vi "format_console_string.vi"(8 "error in (no error)":errorcluster, 11 "log entry":T1 {"datetime" format="%<%x %.3X>T"}) -> (0 "error out":errorcluster, 1 "color":u32, 2 "text":string)   [LabVIEW 2021, in "console.provider.lvclass"]
uses:
  console.provider.lvclass
  system.logging/log_entry.ctl
  system.logging/severity.ctl
  console.provider.lvclass/console.provider.ctl
  system.logging/system.logging.lvclass
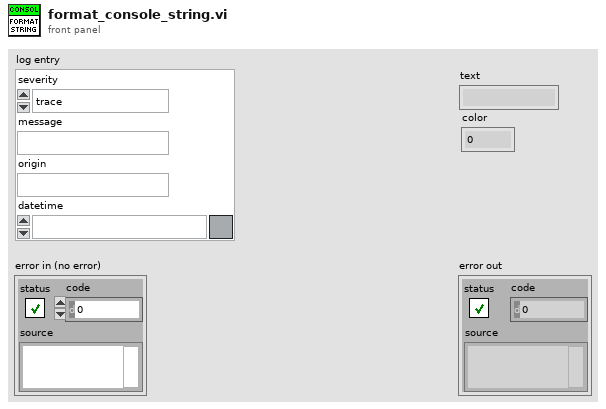
[diagram p1: front panel]
types:
  T1 = typedef "system.logging.lvclass/log_entry.ctl" = cluster{"severity":T2, "message":string, "origin":string, "datetime":timestamp}
  T2 = typedef "system.logging.lvclass/severity.ctl" = enum8{"trace", "debug", "info", "warning", "error"}
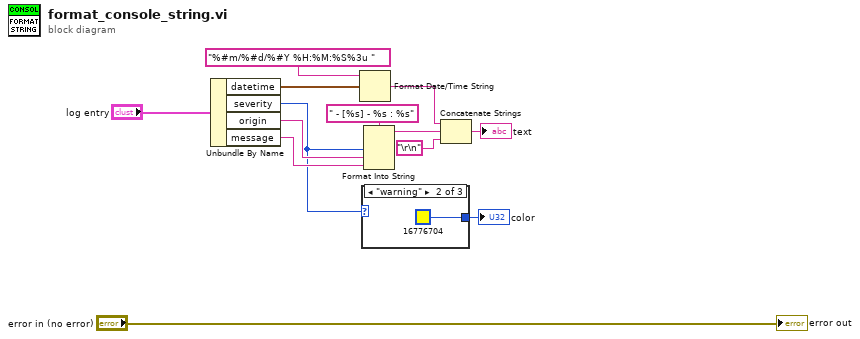
[diagram p0: block diagram]
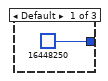
[diagram p2: hidden frame]
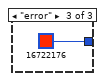
[diagram p3: hidden frame]
diagram:
  n1 = Unbundle By Name("log entry") -> ("datetime"=w11:timestamp, "severity"=w4:T2, "origin"=w10:string, "message"=w9:string)
  n2 = Format Date/Time String(time format string (%c)="%#m/%#d/%#Y %H:%M:%S%3u ", seconds (now)=w11) -> (date/time string=w8:string)  [unwired: 1 in]
  n3 = case shown="\"warning\"" w4 {
    tunnel: [u32 16448250 u32 16776704 u32 16722176] -> w1
    frame Default {
    }
    frame "warning" {
    }
    frame "error" {
    }
  }
  "color" <- w1
  n4 = Format Into String(format string=" - [%s] - %s : %s", w4, w10, w9) -> (resulting string=w7:string)  [unwired: 2 in, 1 out]
  n5 = Concatenate Strings(w8, w7, "\r\n") -> (→"text":string)
  "error out" <- "error in (no error)"
